vi "AlliGator Decay Fit Output String.vi"(0 "Plot Name":string, 1 "(Clipped) Plot Range":T2, 2 "Plot clipped?":bool, 3 "All Fit Parameters":dbl[](array[numeric]), 4 "Guess Parameters Options":T1=enum."User-provided (normalized)", 5 "Fit Output":T3={"best nonlinear fit"=[], "best fit parameters"=[], "R^2"=0.0, "RMSE"=0.0, "error out"={"status"=FALSE, "code"=0, "source"=""}, "Fitting Method"=enum."Least Square", "number of function calls"=0, "number of iterations"=0, "covariance"=[], "Chi 2"=0.0, "DOF"=0, "Fit Convergence Criterion"=enum."Continue", "Fitting Algorithm"=enum."Levenberg-Marquardt", "Weighted Fit"=FALSE, "Gradient"=0.0, "|Delta Chi 2|"=0.0, "|Delta Chi 2|/Chi 2"=0.0, "Max |Delta a| /|a|"=0.0, "Lambda"=-1.0, "RSS"=0.0, "AIC"=0.0, "BIC"=0.0, "Max number of function calls"=0, "Max number of iterations"=0, "IRF"={"X Array"=[], "Y Array"=[]}, "IRF Normalization Factor"=0.0, "Decay Normalization Factor"=0.0}, 7 "Delta Best Fit Parameters":dbl[](array[numeric]), 9 "Fit Options":T9={"Show Fit Residuals"=TRUE, "Fit Model"=enum."1-Exponential", "Residual Type"=enum."Standard", "Max Decay Percentile"=0.0, "Min Decay Percentile"=0.0, "Show Full Decay"=TRUE, "Weights"=enum."Unweighted", "Fitting Method"=enum."Least Square", "Compute Parameter Uncertainties"=TRUE, "Periodic Boundaries"=TRUE, "Model Calculation"=enum."Simulation", "Period"=1.2500000000000001e-08, "Termination Criteria"={"Max Iterations"=1000, "Max Function Calls"=0, "Max Time"=1000.0, "Function Tolerance"=1e-06, "Parameter Tolerance"=1e-06, "Gradient Tolerance"=0.0, "Min Lambda"=1e-06, "Max Lambda"=1e-06, "Initial Tick Count"=0}, "Offset Resolution"=1.2500000000000001e-08, "Use Local IRF"=TRUE, "Fitting Algorithm"=enum."Levenberg-Marquardt"} {"Offset Resolution" min=0.0; "Period" min=0.0; "Min Decay Percentile" min=0.0 max=1.0; "Max Decay Percentile" min=0.0 max=1.0}, 11 "Error In":errorcluster, 12 "Guess Parameters":dbl[](array[numeric]), 13 "Fit Parameter Constraints":T15[](array[typedef]) {"Max Value" format="%#.3g"; "Min Value" format="%#.3g"}, 14 "CPU (s)":dbl) -> (8 "Fit Output Message":string, 15 "Error Out":errorcluster)   [LabVIEW 2021, in "AlliGator Decay Analysis.lvlib" / "AlliGator Decay Fit.lvlib"]
doc: "Creates decay fit output string."
uses:
  AlliGator Decay Fit.lvlib
  AlliGator Decay Fit Parameter Constraints 2.ctl
  Fits/IRF(X)PSED/Decay Fit Parameters In List.ctl
  Fits/IRF(X)PSED/Decay Fit Options v2.ctl
  Fits/Decay Convolution/Decay Model.ctl
  Fits/Residual Type.ctl
  Fits/IRF(X)PSED/Fit Weights Type.ctl
  Fits/Non-linear Fitting Method v2.ctl
  Fits/Fit Calculation Method.ctl
  Fits/Non-linear Fitting Algorithm.ctl
  Fits/Non-linear Fit Output v3.ctl
  Fits/Nonlinear Fit Method.ctl
  <vilib>/Analysis/Matrix/Datatypes/RealMatrix.ctl
  Fits/Convergence Criteria.ctl
  Graphs/XY Graph/XY Plot Data.ctl
  Graphs/Plot Range.ctl
  AlliGator Guess Parameters Options.ctl
  Fits/IRF(X)PSED/Decay Fit Parameters & Derived Quantities List.ctl
  <vilib>/Utility/error.llb/DialogType.ctl
  <vilib>/Utility/error.llb/Error Cluster From Error Code.vi
  <vilib>/ErrorRing/Error Ring.xnode
  Fits/Fits.lvlib
  <vilib>/Analysis/Matrix/NI_Matrix.lvlib
  Graphs/Graphs.lvlib
  Graphs/XY Graph/XY Graph Add-Ons.lvlib
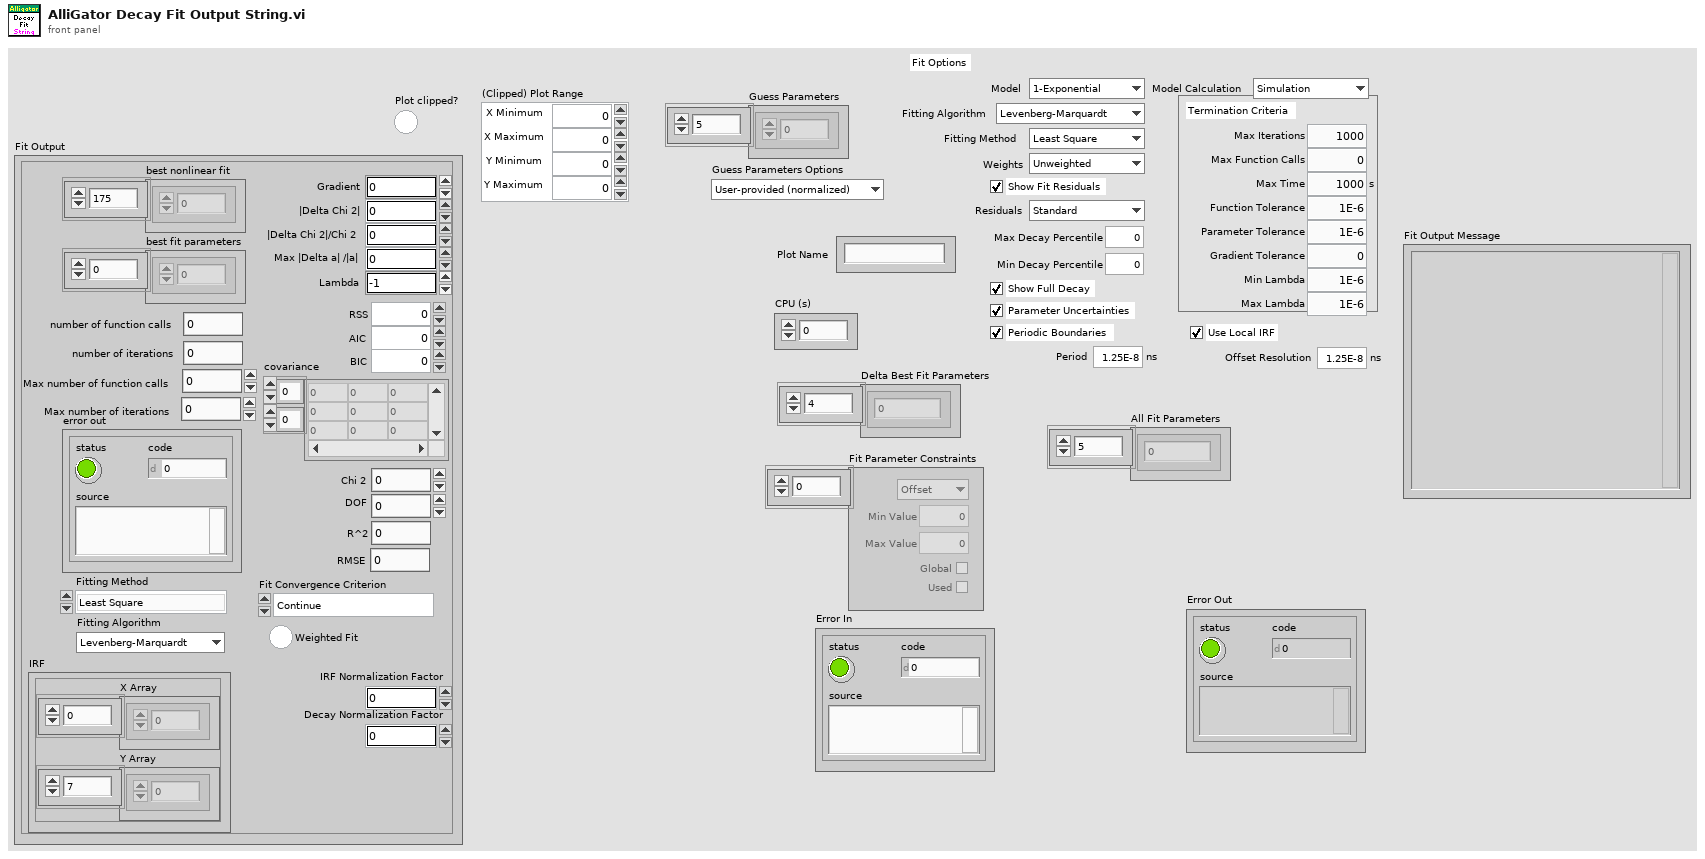
[diagram p1: front panel]
types:
  T1 = typedef "AlliGator Decay Analysis.lvlib/AlliGator Decay Fit.lvlib/AlliGator Guess Parameters Options.ctl" = enum16{"Numerically estimated", "User-provided", "User-provided (normalized)", "Last valid fitted parameters"}
  T2 = typedef "Graphs.lvlib/Plot Range.ctl" = cluster{"X Minimum":dbl, "X Maximum":dbl, "Y Minimum":dbl, "Y Maximum":dbl}
  T3 = typedef "Fits.lvlib/Non-linear Fit Output v3.ctl" = cluster{"best nonlinear fit":dbl[], "best fit parameters":dbl[], "R^2":dbl, "RMSE":dbl, "error out":errorcluster, "Fitting Method":T4, "number of function calls":i32, "number of iterations":i32, "covariance":T5, "Chi 2":dbl, "DOF":i32, "Fit Convergence Criterion":T6, "Fitting Algorithm":T7, "Weighted Fit":bool, "Gradient":dbl, "|Delta Chi 2|":dbl, "|Delta Chi 2|/Chi 2":dbl, "Max |Delta a| /|a|":dbl, "Lambda":dbl, "RSS":dbl, "AIC":dbl, "BIC":dbl, "Max number of function calls":i32, "Max number of iterations":i32, "IRF":T8, "IRF Normalization Factor":dbl, "Decay Normalization Factor":dbl}
  T4 = typedef "Fits.lvlib/Nonlinear Fit Method.ctl" = enum16{"Least Square", "Least Absolute Residual", "Bisquare", "MLE"}
  T5 = typedef "NI_Matrix.lvlib/RealMatrix.ctl" = dbl[][]
  T6 = typedef "Fits.lvlib/Convergence Criteria.ctl" = enum16{"Continue", "Tolerances Exceeded", "Max Time Exceeded", "Max Iterations Exceeded", "Max Function Evaluations Exceeded", "Scale Range Exceeded"}
  T7 = typedef "Fits.lvlib/Non-linear Fitting Algorithm.ctl" = enum16{"Levenberg-Marquardt", "Trust-Region Dogleg"}
  T8 = typedef "XY Graph Add-Ons.lvlib/XY Plot Data.ctl" = cluster{"X Array":dbl[], "Y Array":dbl[]}
  T9 = typedef "Fits.lvlib/Decay Fit Options v2.ctl" = cluster{"Show Fit Residuals":bool, "Fit Model":T10, "Residual Type":T11, "Max Decay Percentile":dbl, "Min Decay Percentile":dbl, "Show Full Decay":bool, "Weights":T12, "Fitting Method":T13, "Compute Parameter Uncertainties":bool, "Periodic Boundaries":bool, "Model Calculation":T14, "Period":dbl[unit], "Termination Criteria":cluster{"Max Iterations":i32, "Max Function Calls":i32, "Max Time":dbl[unit], "Function Tolerance":dbl, "Parameter Tolerance":dbl, "Gradient Tolerance":dbl, "Min Lambda":dbl, "Max Lambda":dbl, "Initial Tick Count":u32}, "Offset Resolution":dbl[unit], "Use Local IRF":bool, "Fitting Algorithm":T7}
  T10 = typedef "Fits.lvlib/Decay Model.ctl" = enum16{"1-Exponential", "2-Exponentials"}
  T11 = typedef "Fits.lvlib/Residual Type.ctl" = enum16{"Standard", "Normalized", "Reduced"}
  T12 = typedef "Fits.lvlib/Fit Weights Type.ctl" = enum16{"Unweighted", "1/Variance", "Best of All"}
  T13 = typedef "Fits.lvlib/Non-linear Fitting Method v2.ctl" = enum16{"Least Square", "Least Absolute Residual", "Bisquare", "MLE", "-", "Best of All"}
  T14 = typedef "Fits.lvlib/Fit Calculation Method.ctl" = enum16{"Simulation", "Convolution", "Integration"}
  T15 = typedef "AlliGator Decay Analysis.lvlib/AlliGator Decay Fit.lvlib/AlliGator Decay Fit Parameter Constraints 2.ctl" = cluster{"Fit Parameter":T16, "Min Value":dbl, "Max Value":dbl, "Global":bool, "Used":bool}
  T16 = typedef "Fits.lvlib/Decay Fit Parameters In List.ctl" = enum16{"Offset", "Baseline", "A_1", "tau_1", "A_2", "tau_2"}
  T17 = cluster{"Max Iterations":i32, "Max Function Calls":i32, "Max Time":dbl[unit], "Function Tolerance":dbl, "Parameter Tolerance":dbl, "Gradient Tolerance":dbl, "Min Lambda":dbl, "Max Lambda":dbl, "Initial Tick Count":u32}
  T18 = typedef "Fits.lvlib/Decay Fit Parameters & Derived Quantities List.ctl" = enum16{"Offset", "Baseline", "A_1", "tau_1", "A_2", "tau_2", "<tau>_a", "f1_a", "f2_a", "<tau>_i", "f1_i", "f2_i", "-", "R^2", "Chi^2"}
  T19 = typedef "DialogType.ctl" = u16
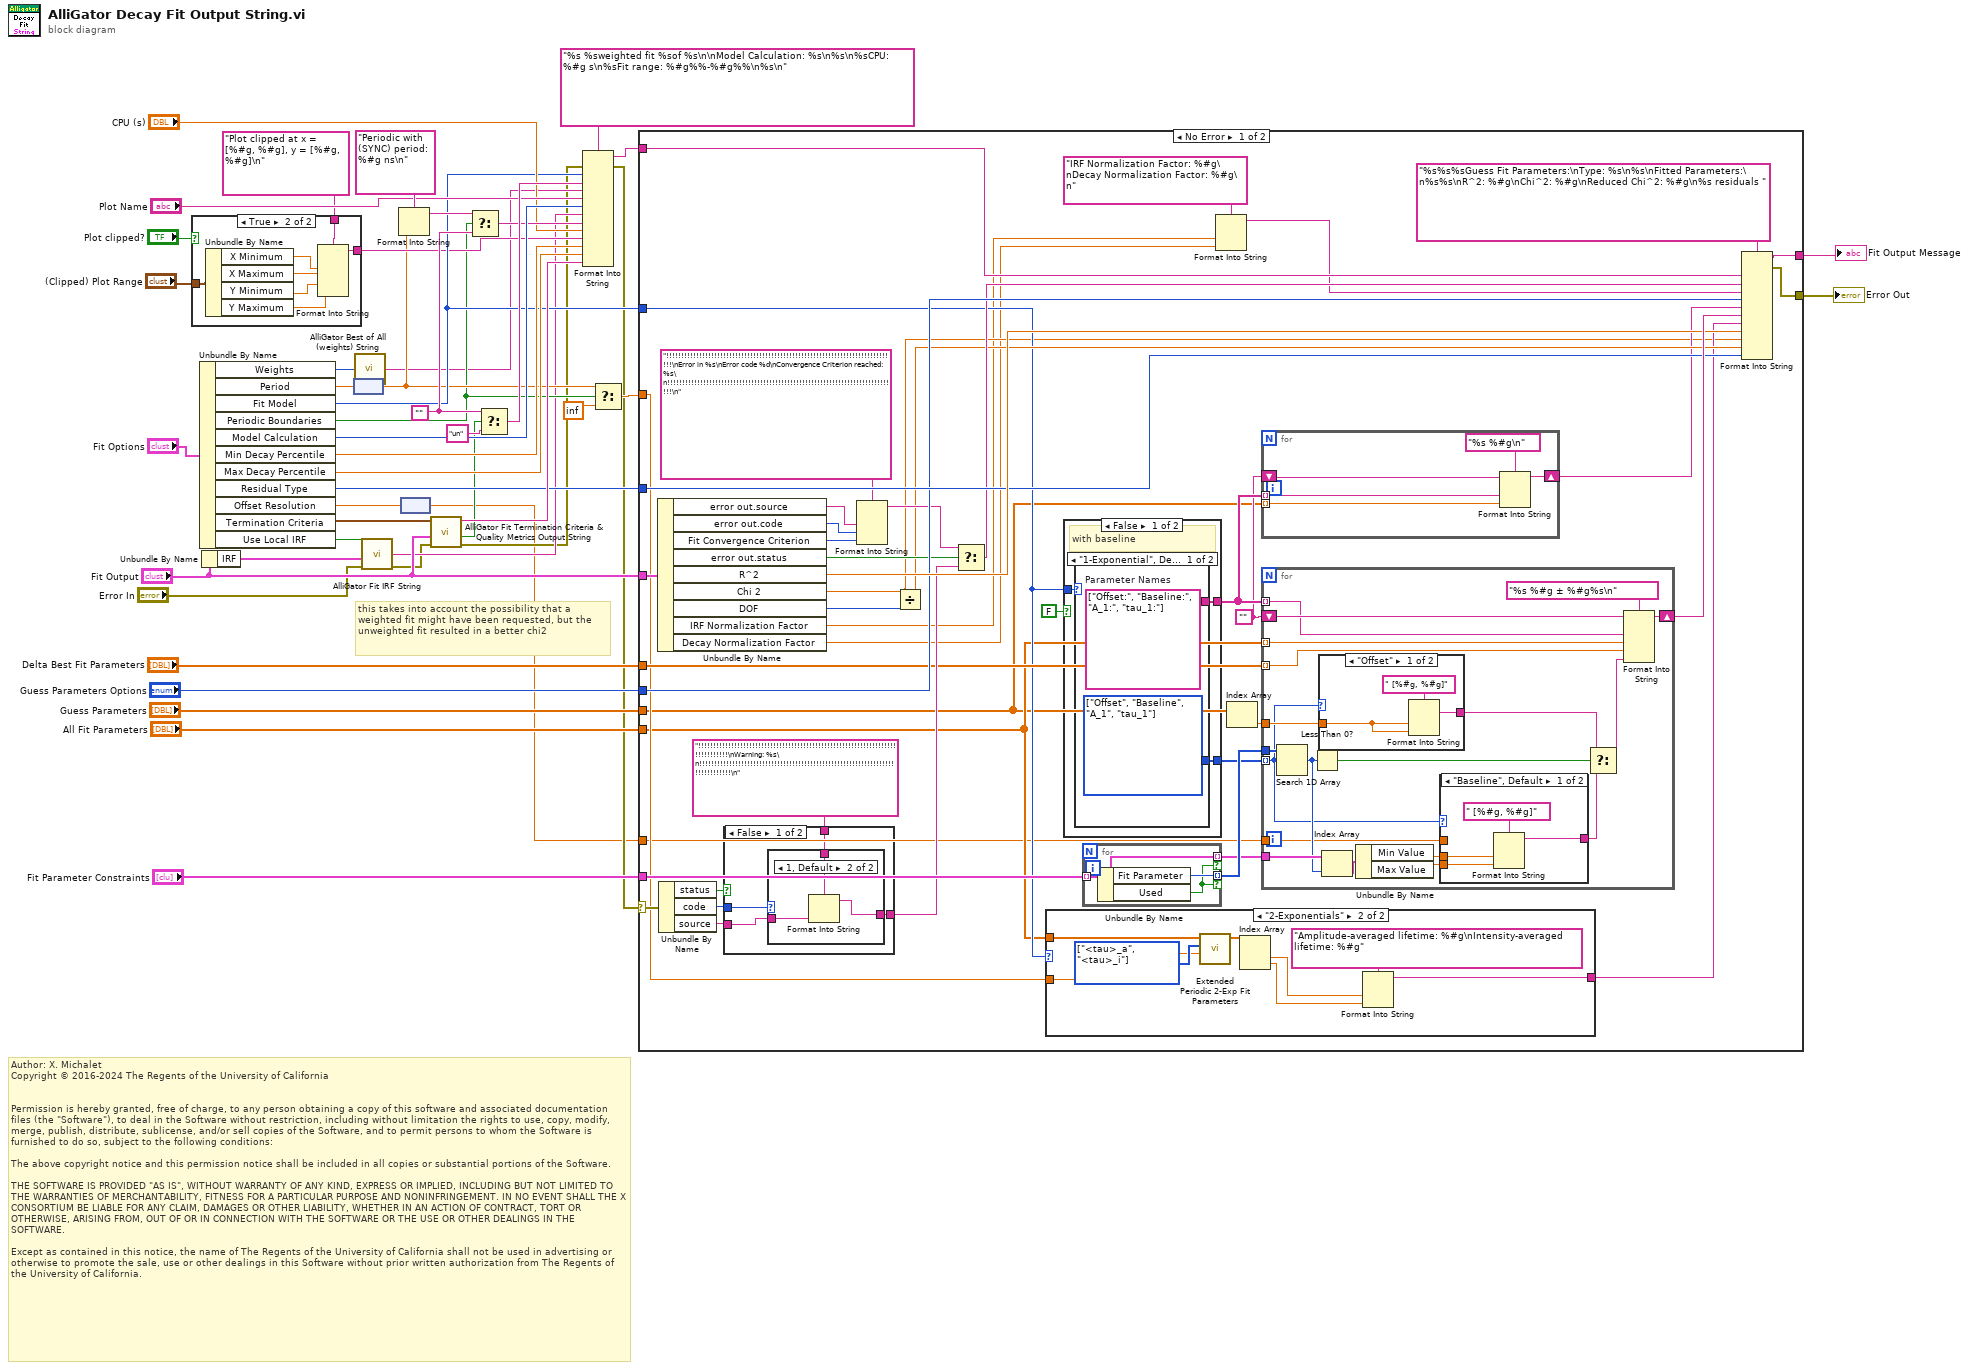
[diagram p0: block diagram]
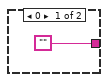
[diagram p4: hidden frame]
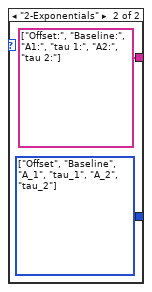
[diagram p6: hidden frame]
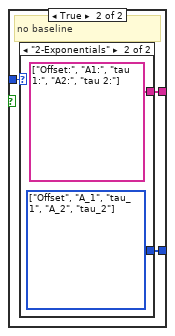
[diagram p7: hidden frame]
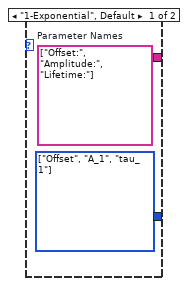
[diagram p8: hidden frame]
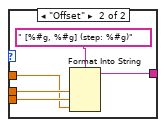
[diagram p9: hidden frame]
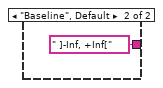
[diagram p10: hidden frame]
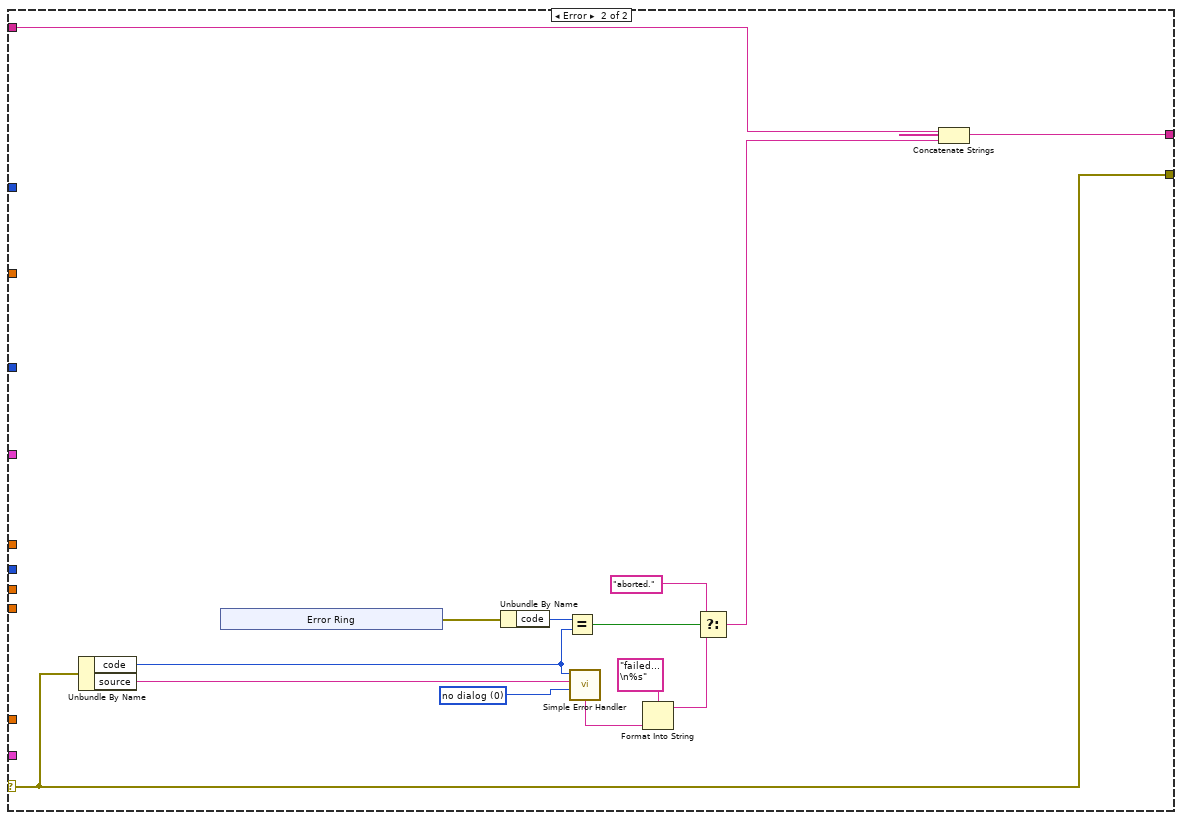
[diagram p11: hidden frame]
diagram:
  w37 = ""
  # "Author: X. Michalet\nCopyright © 2016-2024 The Regents of the University of California\n \n\nPermission is hereby granted, free of charge, to any person obtaining a copy of this software and associated documentation files (the \"Software\"), to deal in the Software without restriction, including without limitation the rights to use, copy, modify, merge, publish, distribute, sublicense, and/or sell copies of the Software, and to permit persons to whom the Software is furnished to do so, subject to the following conditions:\n\nThe above copyright notice and this permission notice shall be included in all copies or substantial portions of the Software.\n\nTHE SOFTWARE IS PROVIDED \"AS IS\", WITHOUT WARRANTY OF ANY KIND, EXPRESS OR IMPLIED, INCLUDING BUT NOT LIMITED TO THE WARRANTIES OF MERCHANTABILITY, FITNESS FOR A PARTICULAR PURPOSE AND NONINFRINGEMENT. IN NO EVENT SHALL THE X CONSORTIUM BE LIABLE FOR ANY CLAIM, DAMAGES OR OTHER LIABILITY, WHETHER IN AN ACTION OF CONTRACT, TORT OR OTHERWISE, ARISING FROM, OUT OF OR IN CONNECTION WITH THE SOFTWARE OR THE USE OR OTHER DEALINGS IN THE SOFTWARE.\n\nExcept as contained in this notice, the name of The Regents of the University of California shall not be used in advertising or otherwise to promote the sale, use or other dealings in this Software without prior written authorization from The Regents of the University of California."
  # "this takes into account the possibility that a weighted fit might have been requested, but the unweighted fit resulted in a better chi2"
  n1 = case shown="True" "Plot clipped?" {
    tunnel: "(Clipped) Plot Range" -> [_ w54]
    tunnel: [_ w49] -> w25
    tunnel: "Plot clipped at x = [%#g, %#g], y = [%#g, %#g]\n" ("format string") -> [_ w48]
    frame False {
    }
    frame True {
      n2 = Unbundle By Name(w54) -> ("X Minimum"=w53:dbl, "X Maximum"=w52:dbl, "Y Minimum"=w51:dbl, "Y Maximum"=w50:dbl)
      n3 = Format Into String(format string=w48, w53, w52, w51, w50) -> (resulting string=w49:string)  [unwired: 2 in, 1 out]
    }
  }
  n4 = Unbundle By Name("Fit Options") -> ("Weights"=w14:T12, "Period"=w15:dbl[unit], "Fit Model"=w29:T10, "Periodic Boundaries"=w16:bool, "Model Calculation"=w38:T14, "Min Decay Percentile"=w33:dbl, "Max Decay Percentile"=w32:dbl, "Residual Type"=w28:T11, "Offset Resolution"=w10:dbl[unit], "Termination Criteria"=w11:T17, "Use Local IRF"=w8:bool)
  n5 = Unbundle By Name("Fit Output") -> ("IRF"=w7:T8)
  n6 = node(w15) -> (w21:dbl)
  n7 = call "AlliGator Best of All (weights) String.vi"("Weights"=w14) -> ("Weights String"=w13:string)
  n8 = call "AlliGator Fit IRF String.vi"("Error In"="Error In", "IRF"=w7, "Use Local IRF"=w8) -> ("Error Out"=w5:errorcluster, "IRF String"=w6:string)  [unwired: 7 in]
  n9 = Format Into String(format string="Periodic with  (SYNC) period: %#g ns\n", w21) -> (resulting string=w36:string)  [unwired: 2 in, 1 out]
  n10 = node(w10) -> (w1:dbl)
  n11 = call "AlliGator Fit Termination Criteria & Quality Metrics Output String.vi"("Error In"=w5, "Fit Output"="Fit Output", "Termination Criteria"=w11) -> ("Error Out"=w4:errorcluster, "Weighted Fit"=w12:bool, "String"=w31:string)  [unwired: 6 in]
  n12 = Select(t=w36, s=w16, f=w37) -> (s? t:f=w35:string)
  n13 = Select(t=w37, s=w12, f="un") -> (s? t:f=w40:string)
  n14 = Format Into String(format string="%s %sweighted fit %sof %s\n\nModel Calculation: %s\n%s\n%sCPU: %#g s\n%sFit range: %#g%%-%#g%%\n%s\n", error in=w4, w29, w40, w13, "Plot Name", w38, w6, w35, "CPU (s)", w25, w33, w32, w31) -> (resulting string=w30:string, error out=w2:errorcluster)  [unwired: 1 in]
  n15 = Select(t=w21, s=w16, f=inf) -> (s? t:f=w19:dbl)
  n16 = case shown="No Error" w2 {
    selector: w2 -> [w93 w170]
    tunnel: "Delta Best Fit Parameters" -> [w70 _]
    tunnel: [w97 w171] -> w46
    tunnel: "Fit Parameter Constraints" -> [w94 _]
    tunnel: "Fit Output" -> [w90 _]
    tunnel: w30 -> [w87 w172]
    tunnel: w29 -> [w66 _]
    tunnel: w28 -> [w86 _]
    tunnel: "Guess Parameters Options" -> [w85 _]
    tunnel: "Guess Parameters" -> [w64 _]
    tunnel: w19 -> [w69 _]
    tunnel: [w67 w170] -> w18
    tunnel: "All Fit Parameters" -> [w65 _]
    tunnel: w1 -> [w59 _]
    frame No Error {
      w72 = ""
      n17 = Unbundle By Name(w90) -> ("error out.source"=w81:string, "error out.code"=w80:i32, "Fit Convergence Criterion"=w76:T6, "error out.status"=w84:bool, "R^2"=w89:dbl, "Chi 2"=w60:dbl, "DOF"=w75:i32, "IRF Normalization Factor"=w56:dbl, "Decay Normalization Factor"=w55:dbl)
      n18 = Unbundle By Name(w93) -> ("status"=w83:bool, "code"=w92:i32, "source"=w91:string)
      n19 = case shown="False" w83 {
        tunnel: w92 -> [w116 _]
        tunnel: w91 -> [w115 _]
        tunnel: [w114 _] -> w82
        tunnel: "!!!!!!!!!!!!!!!!!!!!!!!!!!!!!!!!!!!!!!!!!!!!!!!!!!!!!!!!!!!!!!!!!!!!!!!!!!!!!\nWarning: %s\n!!!!!!!!!!!!!!!!!!!!!!!!!!!!!!!!!!!!!!!!!!!!!!!!!!!!!!!!!!!!!!!!!!!!!!!!!!!!!\n" ("initial string") -> [w113 _]
        frame False {
          n20 = case shown="1, Default" w116 {
            tunnel: ["" w119] -> w114
            tunnel: w115 -> [_ w120]
            tunnel: w113 -> [_ w118]
            frame 0 {
            }
            frame 1, Default {
              n21 = Format Into String(format string=w118, w120) -> (resulting string=w119:string)  [unwired: 2 in, 1 out]
            }
          }
        }
        frame True {
        }
      }
      n22 = Format Into String(format string="!!!!!!!!!!!!!!!!!!!!!!!!!!!!!!!!!!!!!!!!!!!!!!!!!!!!!!!!!!!!!!!!!!!!!!!!!!!!!\nError in %s\nError code %d\nConvergence Criterion reached: %s\n!!!!!!!!!!!!!!!!!!!!!!!!!!!!!!!!!!!!!!!!!!!!!!!!!!!!!!!!!!!!!!!!!!!!!!!!!!!!!\n", w81, w80, w76) -> (resulting string=w79:string)  [unwired: 2 in, 1 out]
      n23 = Divide(x=w60, y=w75) -> (x/y=w74:dbl)
      n24 = Select(t=w79, s=w84, f=w82) -> (s? t:f=w78:string)
      n25 = case shown="\"2-Exponentials\"" w66 {
        tunnel: w69 -> [_ w106]
        tunnel: [_ w101] -> w68
        tunnel: w65 -> [_ w100]
        frame "1-Exponential", Default {
        }
        frame "2-Exponentials" {
          w107 = T18[] [enum."<tau>_a", enum."<tau>_i"] items=["Offset", "Baseline", "A_1", "tau_1", "A_2", "tau_2", "<tau>_a", "f1_a", "f2_a", "<tau>_i", "f1_i", "f2_i", "-", "R^2", "Chi^2"] ("Selected Decay Fit Parameter Array")
          n26 = call "Extended Periodic 2-Exp Fit Parameters.vi"("Laser Period"=w106, "Selected Decay Fit Parameter Array"=w107, "Decay Fit Parameters"=w100) -> ("Extended Decay Fit Parameters"=w105:dbl[])  [unwired: 7 in, 1 out]
          n27 = Index Array(array=w105) -> (element #1=w104:dbl, element #2=w103:dbl)  [unwired: 2 in]
          n28 = Format Into String(format string="Amplitude-averaged lifetime: %#g\nIntensity-averaged lifetime: %#g", w104, w103) -> (resulting string=w101:string)  [unwired: 2 in, 1 out]
        }
      }
      n29 = case shown="False" FALSE {
        tunnel: [w123 w130] -> w73
        tunnel: [w122 w129] -> w95
        tunnel: w66 -> [w121 w128]
        frame False {
          # "with baseline"
          n30 = case shown="\"1-Exponential\", Default" w121 {
            tunnel: [w125 string[] ["Offset:", "Baseline:", "A1:", "tau 1:", "A2:", "tau 2:"] ("Parameter Names")] -> w123
            tunnel: [w124 w126] -> w122
            frame "1-Exponential", Default {
              w124 = T16[] [enum."Offset", enum."Baseline", enum."A_1", enum."tau_1"] items=["Offset", "Baseline", "A_1", "tau_1", "A_2", "tau_2"] ("Array")
              w125 = string[] ["Offset:", "Baseline:", "A_1:", "tau_1:"]  # Parameter Names
            }
            frame "2-Exponentials" {
              w126 = T16[] [enum."Offset", enum."Baseline", enum."A_1", enum."tau_1", enum."A_2", enum."tau_2"] items=["Offset", "Baseline", "A_1", "tau_1", "A_2", "tau_2"] ("Array")
            }
          }
        }
        frame True {
          # "no baseline"
          n31 = case shown="\"2-Exponentials\"" w128 {
            tunnel: [w132 string[] ["Offset:", "A1:", "tau 1:", "A2:", "tau 2:"] ("Parameter Names")] -> w130
            tunnel: [w131 w133] -> w129
            frame "1-Exponential", Default {
              w131 = T16[] [enum."Offset", enum."A_1", enum."tau_1"] items=["Offset", "Baseline", "A_1", "tau_1", "A_2", "tau_2"] ("Array")
              w132 = string[] ["Offset:", "Amplitude:", "Lifetime:"]  # Parameter Names
            }
            frame "2-Exponentials" {
              w133 = T16[] [enum."Offset", enum."A_1", enum."tau_1", enum."A_2", enum."tau_2"] items=["Offset", "Baseline", "A_1", "tau_1", "A_2", "tau_2"] ("Array")
            }
          }
        }
      }
      n32 = for {
        tunnel: w94 -> [w136] mode=indexing
        tunnel: [w137] -> w96 mode=indexing if=w135
        tunnel: [w136] -> w62 mode=indexing if=w135
        n33 = Unbundle By Name(w136) -> ("Fit Parameter"=w137:T16, "Used"=w135:bool)
      }
      n34 = Format Into String(format string="IRF Normalization Factor: %#g\nDecay Normalization Factor: %#g\n", w56, w55) -> (resulting string=w57:string)  [unwired: 2 in, 1 out]
      n35 = Index Array(array=w64) -> (element=w63:dbl)  [unwired: 1 in]
      n36 = for {
        tunnel: w73 -> [w112] mode=indexing
        tunnel: w64 -> [w109] mode=indexing
        shift-right: [w108] -> w71
        shift-left: w72 -> [w110]
        n37 = Format Into String(format string="%s %#g\n", initial string=w110, w112, w109) -> (resulting string=w108:string)  [unwired: 1 in, 1 out]
      }
      n38 = for {
        tunnel: w65 -> [w154] mode=indexing
        tunnel: w70 -> [w153] mode=indexing
        tunnel: w73 -> [w142] mode=indexing
        shift-right: [w156] -> w98
        shift-left: w72 -> [w155]
        tunnel: w96 -> [w151]
        tunnel: w95 -> [w139] mode=indexing
        tunnel: w62 -> [w150]
        tunnel: w63 -> [w140]
        tunnel: w59 -> [w138]
        n39 = Search 1D Array(1D array=w151, element=w139) -> (index of element=w143:i32)  [unwired: 1 in]
        n40 = Less Than 0?(x=w143) -> (x < 0?=w149:bool)
        n41 = case shown="\"Offset\"" w139 {
          tunnel: [w168 " ]-Inf, +Inf[" ("format string")] -> w141
          tunnel: w140 -> [w166 _]
          frame "Offset" {
            n42 = Format Into String(format string=" [%#g, %#g]", w166, w166) -> (resulting string=w168:string)  [unwired: 2 in, 1 out]
          }
          frame "Baseline", Default {
          }
        }
        n43 = Index Array(array=w150, index=w143) -> (element=w147:T15)
        n44 = Unbundle By Name(w147) -> ("Min Value"=w146:dbl, "Max Value"=w145:dbl)
        n45 = case shown="\"Baseline\", Default" w139 {
          tunnel: w146 -> [w159 w165]
          tunnel: w145 -> [w158 w164]
          tunnel: [w157 w162] -> w144
          tunnel: w138 -> [_ w161]
          frame "Baseline", Default {
            n46 = Format Into String(format string=" [%#g, %#g]", w159, w158) -> (resulting string=w157:string)  [unwired: 2 in, 1 out]
          }
          frame "Offset" {
            n47 = Format Into String(format string=" [%#g, %#g] (step: %#g)", w165, w164, w161) -> (resulting string=w162:string)  [unwired: 2 in, 1 out]
          }
        }
        n48 = Select(t=w141, s=w149, f=w144) -> (s? t:f=w148:string)
        n49 = Format Into String(format string="%s %#g ± %#g%s\n", initial string=w155, w142, w154, w153, w148) -> (resulting string=w156:string)  [unwired: 1 in, 1 out]
      }
      n50 = Format Into String(format string="%s%s%sGuess Fit Parameters:\nType: %s\n%s\nFitted Parameters:\n%s%s\nR^2: %#g\nChi^2: %#g\nReduced Chi^2: %#g\n%s residuals ", w87, w78, w57, w85, w71, w98, w68, w89, w60, w74, w86) -> (resulting string=w97:string, error out=w67:errorcluster)  [unwired: 2 in]
    }
    frame Error {
      w177 = T19 0 items=["no dialog", "OK message", "continue or stop message", "OK message + warnings", "continue/stop + warnings"] ("type of dialog (OK msg:1)")
      n51 = Unbundle By Name(w170) -> ("code"=w179:i32, "source"=w178:string)
      n52 = xnode "Error Ring"() -> ("error out"=w183:errorcluster)
      n53 = Unbundle By Name(w183) -> ("code"=w182:i32)
      n54 = Equal?(x=w182, y=w179) -> (x = y?=w181:bool)
      n55 = call <vilib>:"Simple Error Handler.vi"("error code (no error:0)"=w179, "error source (\" \")"=w178, "type of dialog (OK msg:1)"=w177) -> ("message"=w175:string)  [unwired: 2 in, 4 out]
      n56 = Format Into String(format string="failed...\n%s", w175) -> (resulting string=w176:string)  [unwired: 2 in, 1 out]
      n57 = Select(t="aborted." ("input 4"), s=w181, f=w176) -> (s? t:f=w173:string)
      n58 = Concatenate Strings(w172, w173) -> (w171:string)
    }
  }
  "Fit Output Message" <- w46
  "Error Out" <- w18
